vi "Configuration 2.0 JSON Flatten.vi"(8 "error in (no error)":errorcluster, 11 "configuration 2.0":T1={"custom settings"=[], "plugins"=[{"core settings"={"component"="", "values"=[]}, "component settings"=[], "threads"=[{"core settings"={"component"="", "values"=[]}, "component settings"=[], "transfer groups"=[{"core settings"={"component"="Group", "values"=[]}, "component settings"=[], "transfers"=[{"core settings"={"component"="Transfer", "values"=[]}, "component settings"=[], "channels"=[{"core settings"={"component"="Channel", "values"=[]}, "component settings"=[]}]}]}]}]}]}) -> (0 "error out":errorcluster, 2 "dsf version":T2, 3 "dsf configuration json":string)   [LabVIEW 2019, in "DSF Core.lvlib" / "Configuration Session.lvclass"]
uses:
  Configuration Session.lvclass
  Typedefs/DSF Version Info.ctl
  DSF Core.lvlib
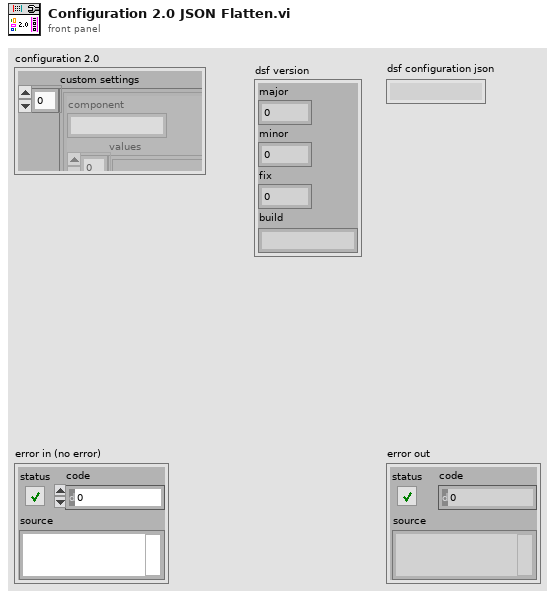
[diagram p1: front panel]
types:
  T1 = cluster{"custom settings":cluster{"component":string, "values":cluster{"key":string, "value":string}[]}[], "plugins":cluster{"core settings":cluster{"component":string, "values":cluster{"key":string, "value":string}[]}, "component settings":cluster{"component":string, "values":cluster{"key":string, "value":string}[]}[], "threads":cluster{"core settings":cluster{"component":string, "values":cluster{"key":string, "value":string}[]}, "component settings":cluster{"component":string, "values":cluster{"key":string, "value":string}[]}[], "transfer groups":cluster{"core settings":cluster{"component":string, "values":cluster{"key":string, "value":string}[]}, "component settings":cluster{"component":string, "values":cluster{"key":string, "value":string}[]}[], "transfers":cluster{"core settings":cluster{"component":string, "values":cluster{"key":string, "value":string}[]}, "component settings":cluster{"component":string, "values":cluster{"key":string, "value":string}[]}[], "channels":cluster{"core settings":cluster{"component":string, "values":cluster{"key":string, "value":string}[]}, "component settings":cluster{"component":string, "values":cluster{"key":string, "value":string}[]}[]}[]}[]}[]}[]}[]}
  T2 = typedef "DSF Core.lvlib/DSF Version Info.ctl" = cluster{"major":u32, "minor":u32, "fix":u32, "build":string}
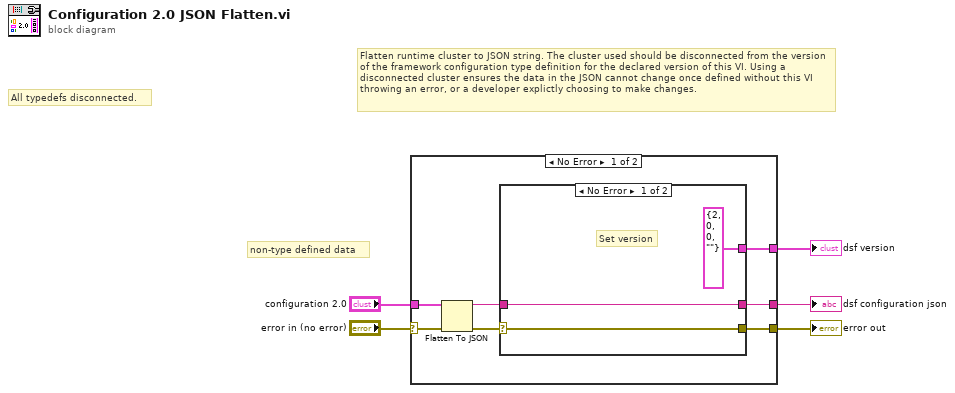
[diagram p0: block diagram]
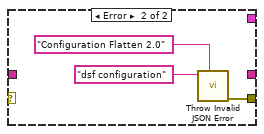
[diagram p2: hidden frame]
diagram:
  # "non-type defined data"
  # "All typedefs disconnected."
  # "Flatten runtime cluster to JSON string. The cluster used should be disconnected from the version of the framework configuration type definition for the declared version of this VI. Using a disconnected cluster ensures the data in the JSON cannot change once defined without this VI throwing an error, or a developer explictly choosing to make changes."
  n1 = case shown="No Error" "error in (no error)" {
    selector: "error in (no error)" -> [w9 w19]
    tunnel: [w11 w19] -> w5
    tunnel: "configuration 2.0" -> [w8 _]
    tunnel: [w7 _] -> w3
    tunnel: [w6 _] -> w2
    frame No Error {
      n2 = Flatten To JSON(anything=w8, error in (no error)=w9) -> (JSON string=w10:string, 11:w12:errorcluster)  [unwired: 1 in]
      n3 = case shown="No Error" w12 {
        selector: w12 -> [w15 _]
        tunnel: [w15 w18] -> w11
        tunnel: w10 -> [w14 _]
        tunnel: [w14 _] -> w7
        tunnel: [T2 {"major"=2, "minor"=0, "fix"=0, "build"=""} ("json version") _] -> w6
        frame No Error {
          # "Set version"
        }
        frame Error {
          n4 = call "Throw Invalid JSON Error.vi"("error source vi name"="Configuration Flatten 2.0", "name"="dsf configuration") -> ("error out"=w18:errorcluster)  [unwired: 9 in]
        }
      }
    }
    frame Error {
    }
  }
  "dsf configuration json" <- w3
  "error out" <- w5
  "dsf version" <- w2
